vi "Create Name Msg.vi"(6 "Name Msg":string, 8 "error in":errorcluster, 9 "Name Library File Path":path, 10 "Active Project":refnum<vi>) -> (0 "error out":errorcluster, 2 "Name Msg":T1)   [LabVIEW 2025, in "_Rescript.lvlib" / "Msg.lvlib" / "Msg.lvclass"]
uses:
  Msg.lvclass
  Msg.lvclass/Msg.ctl
  Name Msg.ctl
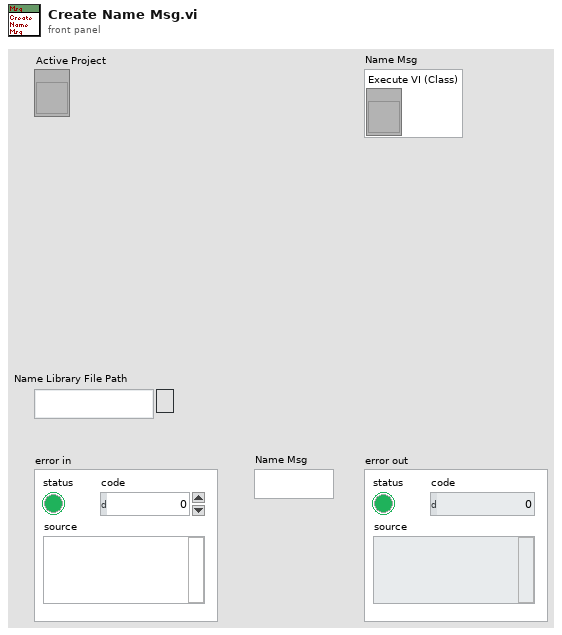
[diagram p1: front panel]
types:
  T1 = typedef "_Rescript.lvlib/Msg.lvlib/Msg.lvclass/Name Msg.ctl" = cluster{"Execute VI (Class)":refnum<vi>}
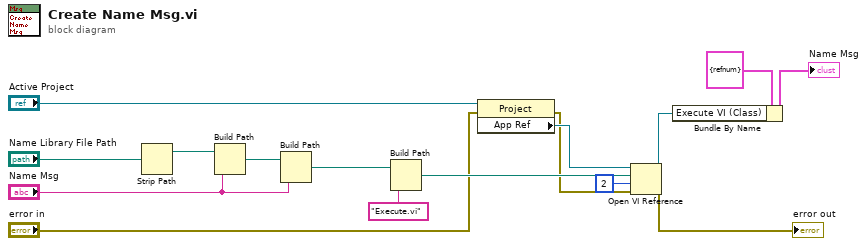
[diagram p0: block diagram]
diagram:
  n1 = Strip Path(path="Name Library File Path") -> (stripped path=w11:path)  [unwired: 1 out]
  n2 = Build Path(base path=w11, name or relative path="Name Msg") -> (appended path=w3:path)
  n3 = Build Path(base path=w3, name or relative path="Name Msg") -> (appended path=w2:path)
  n4 = Build Path(base path=w2, name or relative path="Execute.vi" ("format string")) -> (appended path=w15:path)
  n5 = property class="Project"(reference="Active Project", error in="error in") -> (error out=w1:errorcluster, "App Ref"=w10:refnum<vi>)  [unwired: 1 out]
  n6 = Open VI Reference(application reference (local)=w10, vi path=w15, options=2, error in (no error)=w1) -> (vi reference=w7:refnum<vi>, error out=→"error out":errorcluster)  [unwired: 2 in]
  n7 = Bundle By Name(cluster=T1 {"Execute VI (Class)"=refnum} ("Name Msg Refs"), "Execute VI (Class)"=w7) -> (→"Name Msg":T1)
